vi "Read File.vi"(7 "Section":string, 8 "error in (no error)":errorcluster, 10 "Parameters":refnum<class "Parameter.lvclass">[](array[class]), 11 "Parameter INI File in":refnum<class "Parameter INI File.lvclass">) -> (0 "error out":errorcluster, 2 "Parameters":refnum<class "Parameter.lvclass">[](array[class]), 3 "Parameter INI File out":refnum<class "Parameter INI File.lvclass">)   [LabVIEW 2016, in "CD Parameter Manager API.lvlib" / "Parameter INI File.lvclass"]
uses:
  Parameter INI File.lvclass
  <vilib>/Utility/config.llb/NI_LVConfig.lvlib
  <vilib>/Utility/error.llb/Error Cluster From Error Code.vi
  <vilib>/ErrorRing/Error Ring.xnode
  Boolean Parameter Class/Boolean Parameter.lvclass
  I32 Parameter Class/I32 Parameter.lvclass
  <vilib>/Utility/config.llb/Read Key (Boolean).vi
  <vilib>/Utility/config.llb/Read Key (I32).vi
  Double Parameter Class/Double Parameter.lvclass
  <vilib>/Utility/config.llb/Read Key (Double).vi
  String Parameter Class/String Parameter.lvclass
  <vilib>/Utility/config.llb/Read Key (String).vi
  Parameter Class/Parameter.lvclass
  <vilib>/Utility/config.llb/Read Key (Path).vi
  File Path Parameter Class/File Path Parameter.lvclass
  C:/Repositories/UI-Control-Initializer-API/Source/Parameter Class/Parameter.lvclass
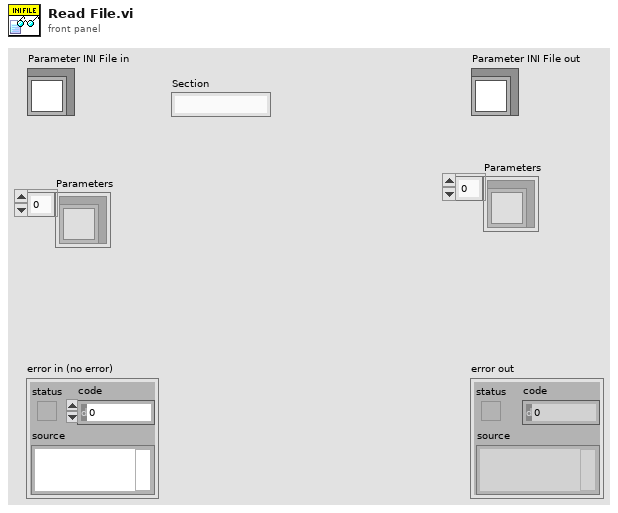
[diagram p1: front panel]
types:
  T1 = typedef "NI_LVConfig.lvlib/Config Data RefNum.ctl" = refnum<k1>
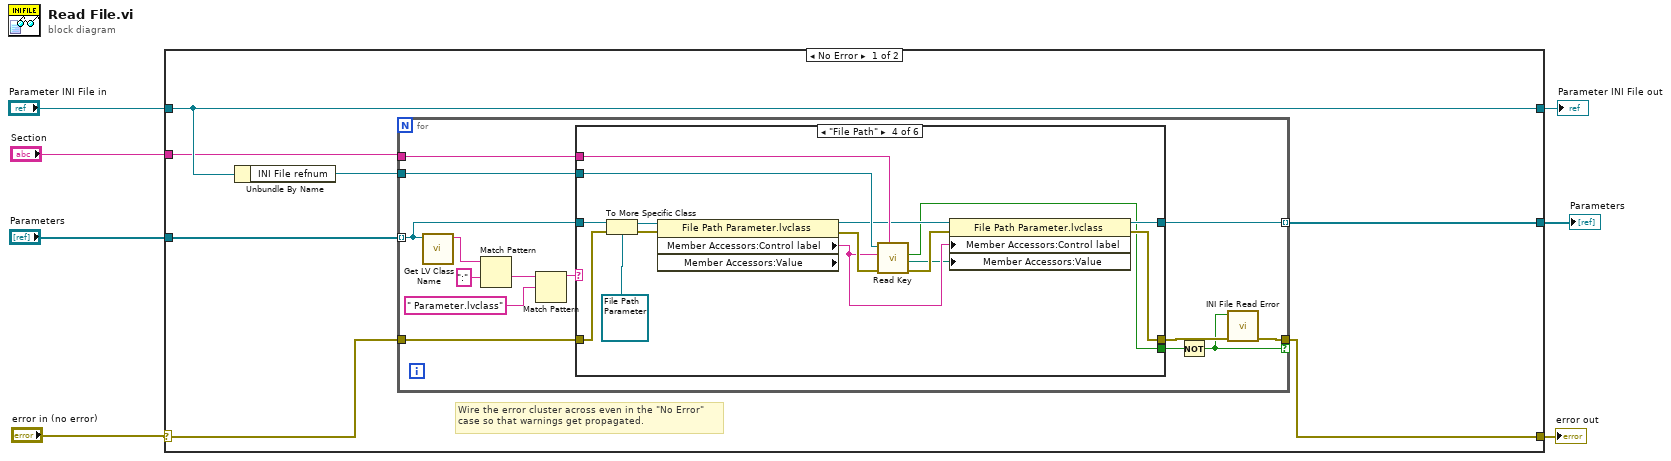
[diagram p0: block diagram]
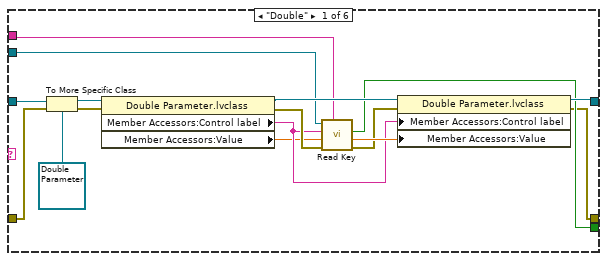
[diagram p2: hidden frame]
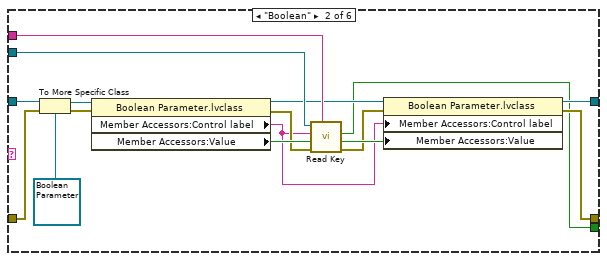
[diagram p3: hidden frame]
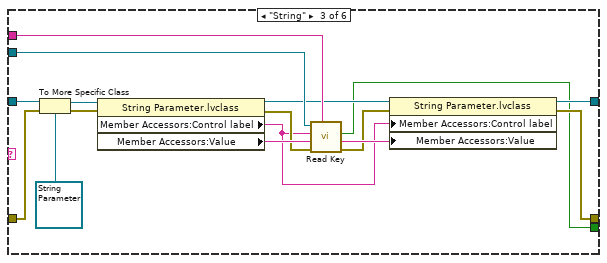
[diagram p4: hidden frame]
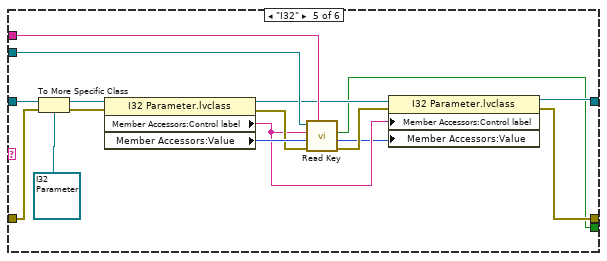
[diagram p5: hidden frame]
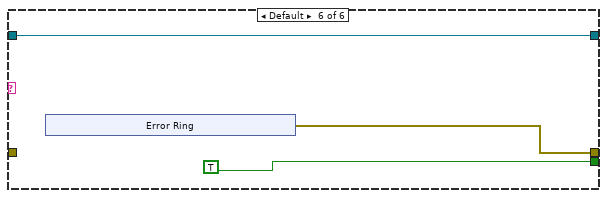
[diagram p6: hidden frame]
diagram:
  n1 = case shown="No Error" "error in (no error)" {
    selector: "error in (no error)" -> [w14 w118]
    tunnel: [w10 w118] -> w5
    tunnel: [w12 w117] -> w6
    tunnel: "Parameter INI File in" -> [w12 w117]
    tunnel: "Parameters" -> [w11 w116]
    tunnel: [w9 w116] -> w2
    tunnel: "Section" -> [w8 _]
    frame No Error {
      # "Wire the error cluster across even in the \"No Error\"\ncase so that warnings get propagated."
      n2 = Unbundle By Name(w12) -> ("INI File refnum"=w13:T1)
      n3 = for {
        tunnel: w14 -> [w23]
        tunnel: [w16] -> w10 if=w15
        tunnel: w13 -> [w21]
        tunnel: w11 -> [w20] mode=indexing
        tunnel: w8 -> [w19]
        tunnel: [w18] -> w9 mode=indexing
        n4 = call <vilib>:"Get LV Class Name.vi"("object"=w20) -> ("class name"=w25:string)  [unwired: 9 in, 1 out]
        n5 = Match Pattern(string=w25, regular expression=":") -> (after substring=w27:string)  [unwired: 1 in, 3 out]
        n6 = Match Pattern(string=w27, regular expression=" Parameter.lvclass") -> (before substring=w24:string)  [unwired: 1 in, 3 out]
        n7 = case shown="\"File Path\"" w24 {
          tunnel: w23 -> [w40 w56 w72 w88 w103 _]
          tunnel: [w31 w47 w64 w81 w94 w109] -> w17
          tunnel: [w32 w45 w62 w79 w92 TRUE] -> w22
          tunnel: w21 -> [w29 w53 w69 w85 w101 _]
          tunnel: w20 -> [w43 w57 w73 w89 w104 w108]
          tunnel: w19 -> [w30 w54 w70 w86 w100 _]
          tunnel: [w33 w46 w63 w80 w97 w108] -> w18
          frame "Double" {
            n8 = To More Specific Class(target class=refnum<class "Double Parameter.lvclass"> refnum ("CD Parameter Manager API.lvlib:Double Parameter.lvclass"), reference=w43, error in=w40) -> (specific class reference=w42:refnum<class "Double Parameter.lvclass">, error out=w44:errorcluster)
            n9 = property class="Double Parameter.lvclass"(reference=w42, error in=w44) -> (reference out=w37:refnum<class "Double Parameter.lvclass">, error out=w36:errorcluster, "Member Accessors:Control label"=w35:string, "Member Accessors:Value"=w34:dbl)
            n10 = call-poly <vilib>:"Read Key.vi"("section"=w30, "error in (no error)"=w36, "default value"=w34, "key"=w35, "refnum"=w29) -> ("error out"=w38:errorcluster, "value"=w39:dbl, "found?"=w32:bool)  [unwired: 3 in, 1 out]
            n11 = property class="Double Parameter.lvclass"(reference=w37, error in=w38, "Member Accessors:Control label"=w35, "Member Accessors:Value"=w39) -> (reference out=w33:refnum<class "Double Parameter.lvclass">, error out=w31:errorcluster)
          }
          frame "Boolean" {
            n12 = To More Specific Class(target class=refnum<class "Boolean Parameter.lvclass"> refnum ("CD Parameter Manager API.lvlib:Boolean Parameter.lvclass"), reference=w57, error in=w56) -> (specific class reference=w59:refnum<class "Boolean Parameter.lvclass">, error out=w60:errorcluster)
            n13 = property class="Boolean Parameter.lvclass"(reference=w59, error in=w60) -> (reference out=w49:refnum<class "Boolean Parameter.lvclass">, error out=w55:errorcluster, "Member Accessors:Control label"=w48:string, "Member Accessors:Value"=w58:bool)
            n14 = call-poly <vilib>:"Read Key.vi"("section"=w54, "error in (no error)"=w55, "default value"=w58, "key"=w48, "refnum"=w53) -> ("error out"=w50:errorcluster, "value"=w51:bool, "found?"=w45:bool)  [unwired: 3 in, 1 out]
            n15 = property class="Boolean Parameter.lvclass"(reference=w49, error in=w50, "Member Accessors:Control label"=w48, "Member Accessors:Value"=w51) -> (reference out=w46:refnum<class "Boolean Parameter.lvclass">, error out=w47:errorcluster)
          }
          frame "String" {
            n16 = To More Specific Class(target class=refnum<class "String Parameter.lvclass"> refnum ("CD Parameter Manager API.lvlib:String Parameter.lvclass"), reference=w73, error in=w72) -> (specific class reference=w75:refnum<class "String Parameter.lvclass">, error out=w76:errorcluster)
            n17 = property class="String Parameter.lvclass"(reference=w75, error in=w76) -> (reference out=w66:refnum<class "String Parameter.lvclass">, error out=w71:errorcluster, "Member Accessors:Control label"=w65:string, "Member Accessors:Value"=w74:string)
            n18 = call-poly <vilib>:"Read Key.vi"("section"=w70, "error in (no error)"=w71, "default value"=w74, "key"=w65, "refnum"=w69) -> ("error out"=w67:errorcluster, "value"=w68:string, "found?"=w62:bool)  [unwired: 3 in, 1 out]
            n19 = property class="String Parameter.lvclass"(reference=w66, error in=w67, "Member Accessors:Control label"=w65, "Member Accessors:Value"=w68) -> (reference out=w63:refnum<class "String Parameter.lvclass">, error out=w64:errorcluster)
          }
          frame "File Path" {
            n20 = To More Specific Class(target class=refnum<class "File Path Parameter.lvclass"> refnum ("CD Parameter Manager API.lvlib:File Path Parameter.lvclass"), reference=w89, error in=w88) -> (specific class reference=w90:refnum<class "File Path Parameter.lvclass">, error out=w91:errorcluster)
            n21 = property class="File Path Parameter.lvclass" props=["Member Accessors:Control label", "Member Accessors:Value"](reference=w90, error in=w91) -> (reference out=w83:refnum<class "File Path Parameter.lvclass">, error out=w87:errorcluster, "Member Accessors:Control label"=w82:string)  [unwired: 1 out]
            n22 = call-poly <vilib>:"Read Key.vi"("section"=w86, "error in (no error)"=w87, "key"=w82, "refnum"=w85) -> ("error out"=w84:errorcluster, "value"=w77:path, "found?"=w79:bool)  [unwired: 4 in, 1 out]
            n23 = property class="File Path Parameter.lvclass"(reference=w83, error in=w84, "Member Accessors:Control label"=w82, "Member Accessors:Value"=w77) -> (reference out=w80:refnum<class "File Path Parameter.lvclass">, error out=w81:errorcluster)
          }
          frame "I32" {
            n24 = To More Specific Class(target class=refnum<class "I32 Parameter.lvclass"> refnum ("CD Parameter Manager API.lvlib:I32 Parameter.lvclass"), reference=w104, error in=w103) -> (specific class reference=w106:refnum<class "I32 Parameter.lvclass">, error out=w107:errorcluster)
            n25 = property class="I32 Parameter.lvclass"(reference=w106, error in=w107) -> (reference out=w98:refnum<class "I32 Parameter.lvclass">, error out=w102:errorcluster, "Member Accessors:Control label"=w95:string, "Member Accessors:Value"=w105:i32)
            n26 = call-poly <vilib>:"Read Key.vi"("section"=w100, "error in (no error)"=w102, "default value"=w105, "key"=w95, "refnum"=w101) -> ("error out"=w96:errorcluster, "value"=w93:i32, "found?"=w92:bool)  [unwired: 3 in, 1 out]
            n27 = property class="I32 Parameter.lvclass"(reference=w98, error in=w96, "Member Accessors:Control label"=w95, "Member Accessors:Value"=w93) -> (reference out=w97:refnum<class "I32 Parameter.lvclass">, error out=w94:errorcluster)
          }
          frame Default {
            n28 = xnode "Error Ring"() -> ("error out"=w109:errorcluster)
          }
        }
        n29 = Not(x=w22) -> (.not. x?=w15:bool)
        n30 = call "INI File Read Error.vi"("error in (no error)"=w17, "INI Key Not Found?"=w15) -> ("error out"=w16:errorcluster)  [unwired: 9 in]
      }
    }
    frame Error {
    }
  }
  "error out" <- w5
  "Parameter INI File out" <- w6
  "Parameters" <- w2
